vi "Gen_ctrl.vi"(8 "error in (no error)":errorcluster, 9 "Controller On?":bool, 10 "Kp":dbl=1.0, 11 "Error In":dbl) -> (0 "error out":errorcluster, 3 "Ctrl Effort Out":dbl)   [LabVIEW 2016, in "Controller.lvlib"]
doc: "Generic Continuous time controller"
uses:
  Controller.lvlib
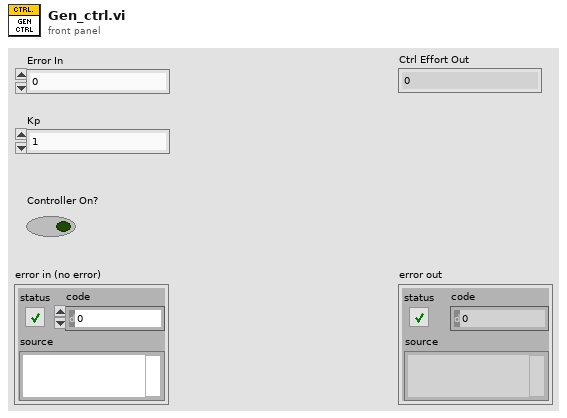
[diagram p1: front panel]
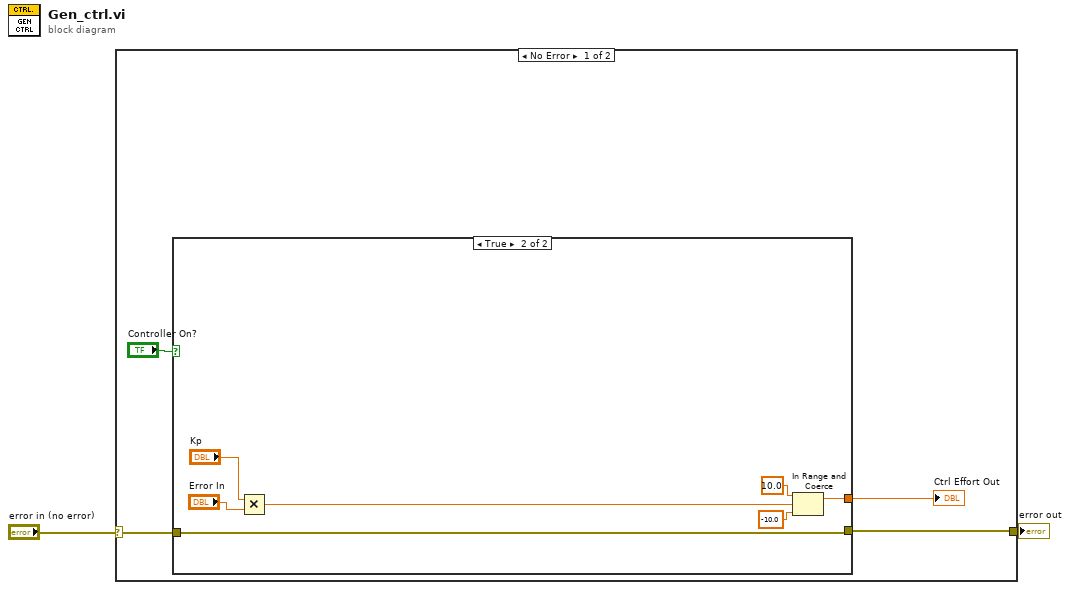
[diagram p0: block diagram]
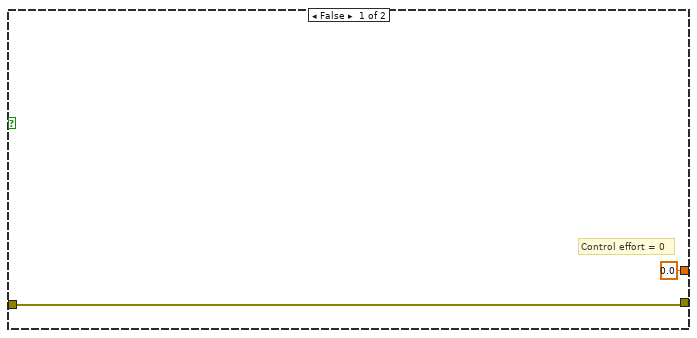
[diagram p2: hidden frame]
diagram:
  n1 = case shown="No Error" "error in (no error)" {
    selector: "error in (no error)" -> [w6 w16]
    tunnel: [w5 w16] -> w1
    frame No Error {
      n2 = case shown="True" "Controller On?" {
        tunnel: w6 -> [w7 w13]
        tunnel: [w7 w13] -> w5
        tunnel: [0.0 ("upper limit") w12] -> w3
        frame False {
          # "Control effort = 0"
        }
        frame True {
          n3 = Multiply(x="Kp", y="Error In") -> (x*y=w11:dbl)
          n4 = In Range and Coerce(upper limit=10.0, x=w11, lower limit=-10.0) -> (coerced(x)=w12:dbl)  [unwired: 1 out]
        }
      }
      "Ctrl Effort Out" <- w3
    }
    frame Error {
    }
  }
  "error out" <- w1
